vi "Name file.vi"(9 "Time Stamp":timestamp, 10 "Test Name":string, 11 "Folder Location":path) -> (3 "Generated File Path":path)   [LabVIEW 2020]
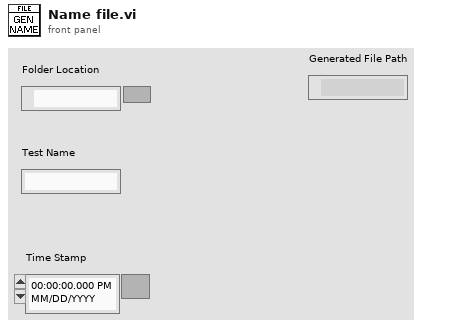
[diagram p1: front panel]
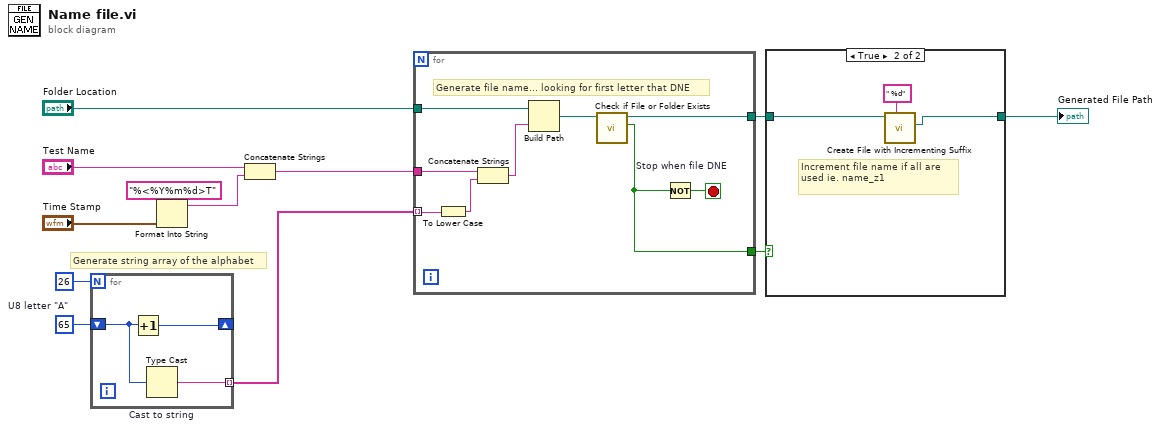
[diagram p0: block diagram]
diagram:
  w12 = u8 65  # U8 letter "A"
  # "Generate string array of the alphabet"
  n1 = for {
    N: 26 -> [_]
    shift-right: [w15] -> _
    shift-left: w12 -> [w14]
    tunnel: [w13] -> w10 mode=indexing
    n2 = Increment(x=w14) -> (x+1=w15:u8)
    n3 = Type Cast "Cast to string"(x=w14) -> (*(type *) &x=w13:string)  [unwired: 1 in]
  }
  n4 = Format Into String(format string="%<%Y%m%d>T", "Time Stamp") -> (resulting string=w6:string)  [unwired: 2 in, 1 out]
  n5 = Concatenate Strings("Test Name", w6) -> (w2:string)
  n6 = for {
    tunnel: "Folder Location" -> [w24]
    tunnel: w10 -> [w23] mode=indexing
    tunnel: [w20] -> w4
    tunnel: [w17] -> w3
    tunnel: w2 -> [w16]
    stop <- w18 stop-if-true
    # "Generate file name... looking for first letter that DNE"
    n7 = To Lower Case(string=w23) -> (all lower case string=w19:string)
    n8 = Concatenate Strings(w16, w19) -> (w22:string)
    n9 = Build Path(base path=w24, name or relative path=w22) -> (appended path=w21:path)
    n10 = call <vilib>:"Check if File or Folder Exists.vi"("path"=w21) -> ("file or folder exists?"=w17:bool, "dup path"=w20:path)  [unwired: 8 in, 1 out]
    n11 = Not "Stop when file DNE"(x=w17) -> (.not. x?=w18:bool)
  }
  n12 = case shown="True" w3 {
    tunnel: [w25 w27] -> w5
    tunnel: w4 -> [w25 w26]
    frame False {
    }
    frame True {
      # "Increment file name if all are used ie. name_z1"
      n13 = call <vilib>:"Create File with Incrementing Suffix.vi"("format string (\" (%d)\")"=" %d" ("format string (\" (%d)\")"), "file path"=w26) -> ("actual path"=w27:path)  [unwired: 7 in, 2 out]
    }
  }
  "Generated File Path" <- w5
